vi "Create Point by X and Y.vi"(8 "error in (no error)":errorcluster caption="错误输入（无错误）", 10 "Y":dbl, 11 "X":dbl) -> (0 "error out":errorcluster caption="错误输出", 3 "Point 输出":refnum<class "Point.lvclass"> caption="DNL_LabVIEW Object out")   [LabVIEW 2011, in "Point.lvclass"]
uses:
  Point.lvclass
  Point.lvclass/Point.ctl
panel:
  in  "Point 输入":refnum<class "Point.lvclass"> caption="DNL_LabVIEW Object in"
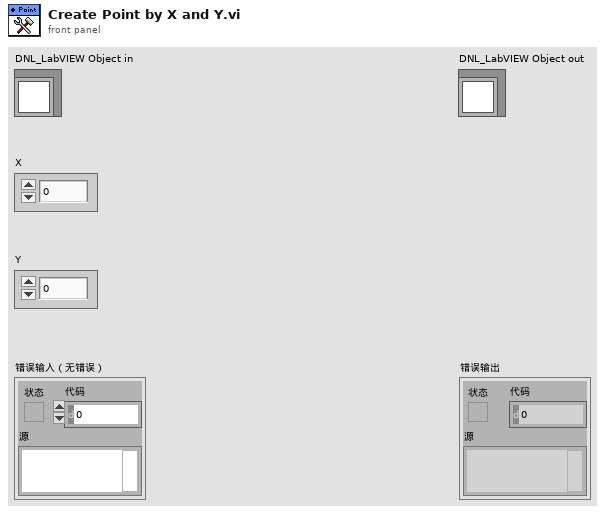
[diagram p1: front panel]
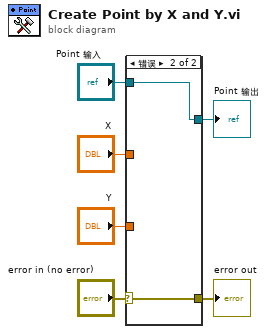
[diagram p0: block diagram]
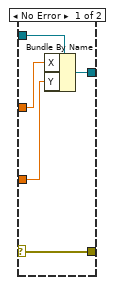
[diagram p2: hidden frame]
diagram:
  n1 = case shown="错误" "error in (no error)" {
    selector: "error in (no error)" -> [w11 w13]
    tunnel: [w11 w13] -> w5
    tunnel: [w7 w12] -> w3
    tunnel: "Point 输入" -> [w10 w12]
    tunnel: "X" -> [w9 _]
    tunnel: "Y" -> [w8 _]
    frame No Error {
      n2 = Bundle By Name(cluster=w10, "X"=w9, "Y"=w8) -> (w7:refnum<class "Point.lvclass">)
    }
    frame Error {
    }
  }
  "error out" <- w5
  "Point 输出" <- w3
